vi "Home.vi"(8 "error in (no error)":errorcluster, 9 "Interlock Chain":refnum<class "Interlock Chain.lvclass">, 11 "Cylinder in":refnum<class "Cylinder.lvclass">) -> (0 "error out":errorcluster, 3 "Cylinder out":refnum<class "Cylinder.lvclass">)   [LabVIEW 2015, in "cRIO-Carbondioxide.lvlib" / "CO2-Actor.lvlib" / "Cylinder.lvclass"]
uses:
  Cylinder.lvclass
  Interlocks/Interlock Chain/Interlock Chain.lvclass
  <vilib>/ActorFramework/Actor/Actor.lvclass/Actor.ctl
  <vilib>/ActorFramework/Message Enqueuer/Message Enqueuer.lvclass/Message Enqueuer.ctl
  Cylinder.lvclass/Cylinder.ctl
  <vilib>/ActorFramework/Actor/Read Self Enqueuer.vi
  <vilib>/ActorFramework/Message Enqueuer/Init from Existing Queue.vi
  <vilib>/ActorFramework/Actor/Actor.lvclass
  <vilib>/ActorFramework/Message Enqueuer/Message Enqueuer.lvclass
  CO2 Actor/CO2 Actor.lvclass
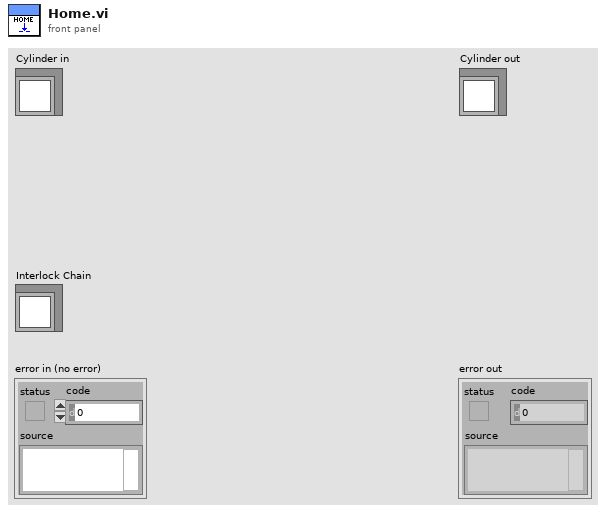
[diagram p1: front panel]
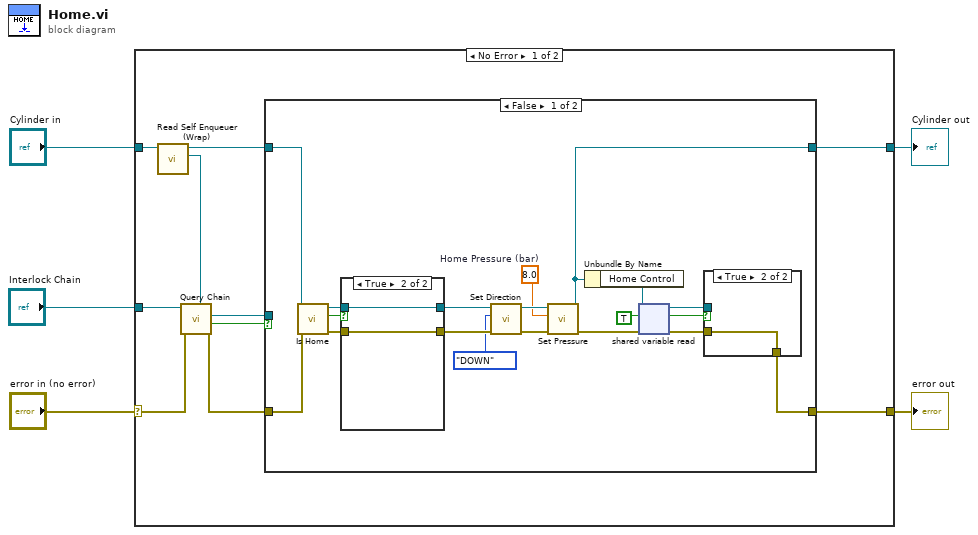
[diagram p0: block diagram]
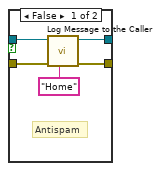
[diagram p2: hidden frame]
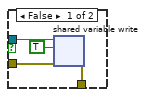
[diagram p3: hidden frame]
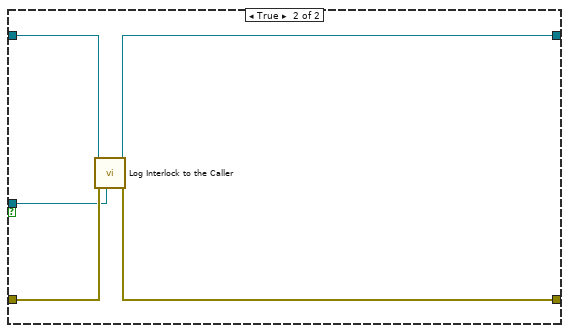
[diagram p4: hidden frame]
diagram:
  n1 = case shown="No Error" "error in (no error)" {
    selector: "error in (no error)" -> [w14 w53]
    tunnel: [w12 w53] -> w4
    tunnel: [w13 w52] -> w2
    tunnel: "Cylinder in" -> [w8 w52]
    tunnel: "Interlock Chain" -> [w15 _]
    frame No Error {
      n2 = call "Read Self Enqueuer (Wrap).vi"("CO2 Actor in"=w8) -> ("Actor Framework:Message Enqueuer"=w6:refnum<class "Message Enqueuer.lvclass">, "CO2 Actor out"=w7:refnum<class "Cylinder.lvclass">)  [unwired: 9 in]
      n3 = call "Query Chain.vi"("Caller Enqueuer"=w6, "error in (no error)"=w14, "Interlock Chain"=w15) -> ("error out"=w9:errorcluster, "Interlock?"=w10:bool, "Interlock out"=w11:refnum<class "Interlock.lvclass">)  [unwired: 3 in, 3 out]
      n4 = case shown="False" w10 {
        tunnel: w7 -> [w20 w51]
        tunnel: [w26 w48] -> w13
        tunnel: w9 -> [w18 w50]
        tunnel: [w21 w47] -> w12
        tunnel: w11 -> [_ w49]
        frame False {
          w30 = 8.0  # Home Pressure (bar)
          n5 = call "Is Home.vi"("error in (no error)"=w18, "Cylinder in"=w20) -> ("error out"=w17:errorcluster, "Cylinder is Home"=w16:bool, "Cylinder out"=w19:refnum<class "Cylinder.lvclass">)  [unwired: 6 in, 1 out]
          n6 = case shown="True" w16 {
            tunnel: [w39 w41] -> w34
            tunnel: [w38 w40] -> w33
            tunnel: w19 -> [w36 w41]
            tunnel: w17 -> [w35 w40]
            frame False {
              # "Antispam"
              n7 = call-dynamic "Log Message to the Caller.vi"("String (\"\" = no message to send)"="Home" ("String (\"\" = no message to send)"), "error in (no error)"=w35, "CO2 Actor in"=w36) -> ("error out"=w38:errorcluster, "CO2 Actor out"=w39:refnum<class "Cylinder.lvclass">)  [unwired: 7 in]
            }
            frame True {
            }
          }
          n8 = call "Set Direction.vi"("error in (no error)"=w33, "Direction (Down)"=enum16{"UP", "DOWN"}."DOWN", "Cylinder in"=w34) -> ("error out"=w32:errorcluster, "Cylinder out"=w31:refnum<class "Cylinder.lvclass">)  [unwired: 7 in]
          n9 = call "Set Pressure.vi"("error in (no error)"=w32, "Pressure (bar)"=w30, "Cylinder in"=w31) -> ("error out"=w22:errorcluster, "Cylinder out"=w26:refnum<class "Cylinder.lvclass">)  [unwired: 7 in]
          n10 = Unbundle By Name(w26) -> ("Home Control"=w28:refnum<k21>)
          n11 = shared-variable-read(w28, w22, TRUE) -> (w24:refnum<k21>, w25:errorcluster, w23:bool)  [unwired: 1 out]
          n12 = case shown="True" w23 {
            tunnel: w25 -> [w45 w46]
            tunnel: w24 -> [w44 _]
            tunnel: [w42 w46] -> w21
            frame False {
              n13 = shared-variable-write(w44, w45, TRUE ("data in")) -> (w42:errorcluster)  [unwired: 1 out]
            }
            frame True {
            }
          }
        }
        frame True {
          n14 = call-dynamic "Log Interlock to the Caller.vi"("Interlock in"=w49, "error in (no error)"=w50, "CO2 Actor in"=w51) -> ("error out"=w47:errorcluster, "CO2 Actor out"=w48:refnum<class "Cylinder.lvclass">)  [unwired: 7 in]
        }
      }
    }
    frame Error {
    }
  }
  "error out" <- w4
  "Cylinder out" <- w2
